vi "Set Steer Motors.vi"(5 "Disable":bool, 6 "PPR":dbl=1024.0, 7 "Offset Encoder Positions":dbl[](array[numeric]), 8 "Steer Control Mode":T2, 9 "Motor List":T1[](array[typedef])=[enum."Right-Front", enum."Left-Front", enum."Left-Back", enum."Right-Back"], 10 "Swerve Data":T8 {"Back Right"."Angle" scale format="%.3f"; "Back Right"."Velocity" scale=-1.0..1.0 scale format="%.1f"; "Back Left"."Angle" scale format="%.3f"; "Back Left"."Velocity" scale=-1.0..1.0 scale format="%.1f"; "Front Left"."Angle" scale format="%.3f"; "Front Left"."Velocity" scale=-1.0..1.0 scale format="%.1f"; "Front Right"."Angle" scale format="%.3f"; "Front Right"."Velocity" scale=-1.0..1.0 scale format="%.1f"}, 11 "Steer Refs":T3[](array[typedef])) -> (1 "Encoder Counts Out":dbl[](array[numeric]), 3 "Array Out":T3[](array[typedef]))   [LabVIEW 2023, in "SwerveDrive_ACT_ts.lvlib"]
uses:
  SwerveDrive_ACT_ts.lvlib
  Shared Code/TypeDefs/Cluster_Swerve 4 Steer and Velocity.ctl
  Shared Code/TypeDefs/Cluster_Module Velocity-Direction-Rotations.ctl
  Shared Code/TypeDefs/Level_Velocity plus-minus 1.ctl
  Shared Code/TypeDefs/Dial_Compase heading unit circle CCW positive.ctl
  <vilib>/Rock Robotics/WPI/MotorControl/WPI_MotorControlDeviceRef.ctl
  <vilib>/Rock Robotics/WPI/MotorControl/WPI_MotorControlType.ctl
  <vilib>/Rock Robotics/SystemInterfaces/DIO/FPGA_DIOPWMChannel.ctl
  <vilib>/Rock Robotics/WPI/PWM/WPI_PWMDeadband.ctl
  <vilib>/Rock Robotics/SystemInterfaces/DIO/FPGA_DIOChannel.ctl
  Type Defs/ENUM_Steer Mode Select.ctl
  Shared Code/TypeDefs/ENUM_Module Position.ctl
  <vilib>/Rock Robotics/WPI/ThirdParty/REV Robotics/REVLib/Typedef/Spark MAX Control Type.ctl
panel:
  # "\"Front\" of Robot"
  # "Index 1"
  # "Index 0"
  # "Index 3"
  # "Index 2"
  # "Right Hand Rule"
  # "X"
  # "+CCW"
  # "Y"
  # "(0,0)"
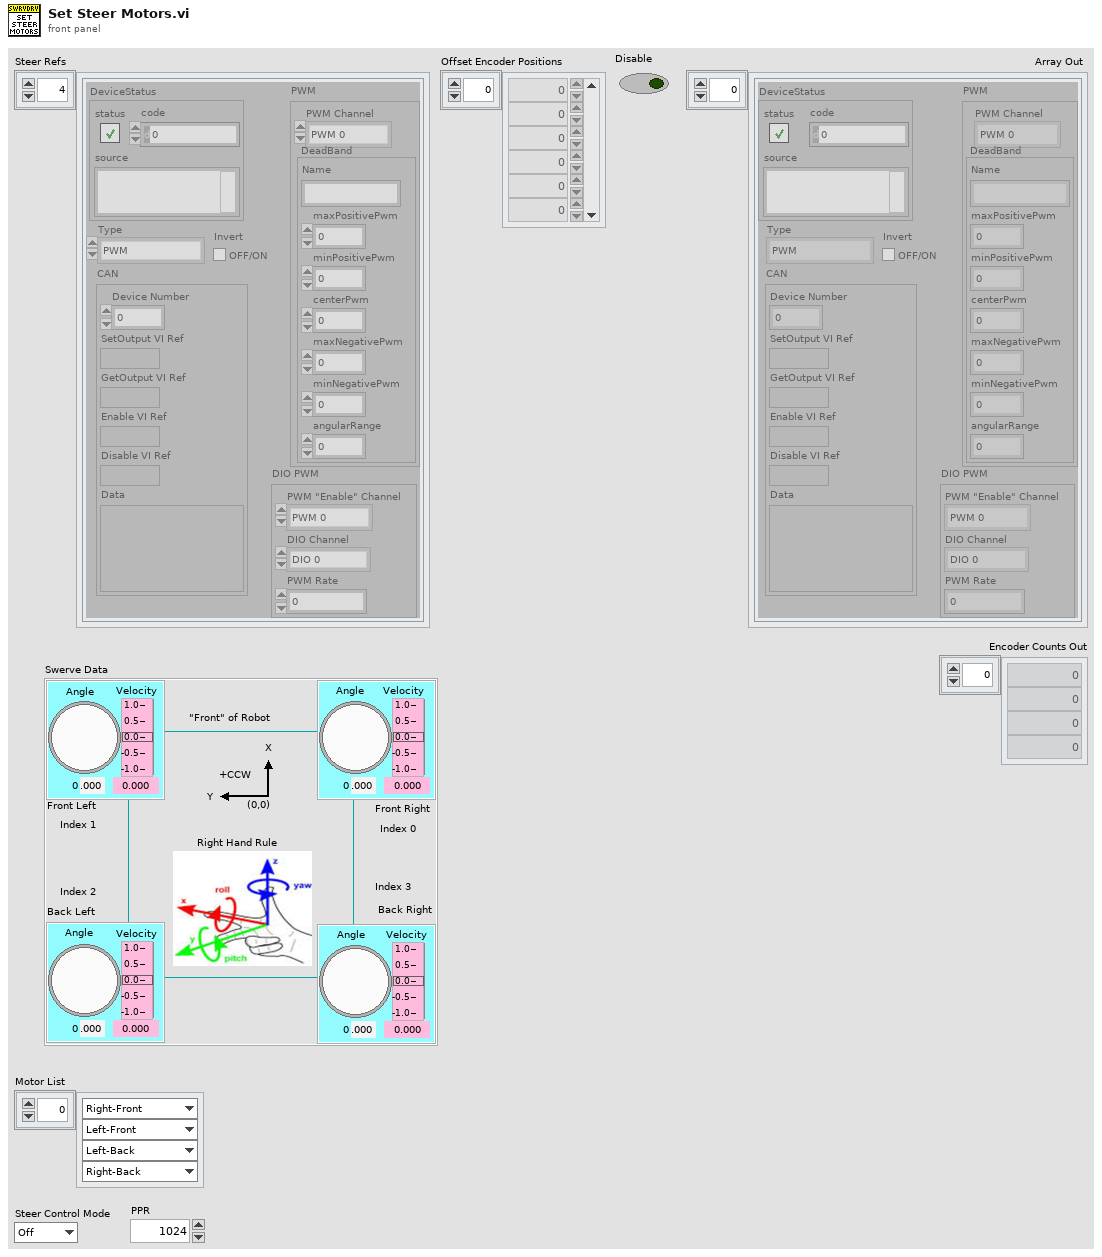
[diagram p1: front panel]
types:
  T1 = typedef "ENUM_Module Position.ctl" = enum16{"Left-Front", "Right-Front", "Left-Back", "Right-Back"}
  T2 = typedef "ENUM_Steer Mode Select.ctl" = enum16{"Off", "Hold", "Steer"}
  T3 = typedef "WPI_MotorControlDeviceRef.ctl" = cluster{"DeviceStatus":errorcluster, "Type":T4, "PWM":cluster{"PWM Channel":T5, "DeadBand":T6}, "CAN":cluster{"Device Number":u8, "SetOutput VI Ref":variant, "GetOutput VI Ref":variant, "Enable VI Ref":variant, "Disable VI Ref":variant, "Data":variant}, "Invert":bool, "DIO PWM":cluster{"PWM \"Enable\" Channel":T5, "DIOChannel":T7, "PWM Rate":dbl}}
  T4 = typedef "WPI_MotorControlType.ctl" = enum16{"PWM", "CAN", "DIO PWM"}
  T5 = typedef "FPGA_DIOPWMChannel.ctl" = enum8{"PWM 0", "PWM 1", "PWM 2", "PWM 3", "PWM 4", "PWM 5", "PWM 6", "PWM 7", "PWM 8", "PWM 9", "PWM MXP 0", "PWM MXP 1", "PWM MXP 2", "PWM MXP 3", "PWM MXP 4", "PWM MXP 5", "PWM MXP 6", "PWM MXP 7", "PWM MXP 8", "PWM MXP 9", "Invalid"}
  T6 = typedef "WPI_PWMDeadband.ctl" = cluster{"Name":string, "maxPositivePwm":i32, "minPositivePwm":i32, "centerPwm":i32, "maxNegativePwm":i32, "minNegativePwm":i32, "angularRange":u16}
  T7 = typedef "FPGA_DIOChannel.ctl" = enum8{"DIO 0", "DIO 1", "DIO 2", "DIO 3", "DIO 4", "DIO 5", "DIO 6", "DIO 7", "DIO 8", "DIO 9", "DIO MXP 0", "DIO MXP 1", "DIO MXP 2", "DIO MXP 3", "DIO MXP 4", "DIO MXP 5", "DIO MXP 6", "DIO MXP 7", "DIO MXP 8", "DIO MXP 9", "DIO MXP 10", "DIO MXP 11", "DIO MXP 12", "DIO MXP 13", "DIO MXP 14", "DIO MXP 15", "SPI Port CS1", "SPI Port CS2", "SPI Port CS3", "SPI Port MISO", "SPI Port MOSI", "Invalid"}
  T8 = typedef "Cluster_Swerve 4 Steer and Velocity.ctl" = cluster{"Front Right":T9, "Front Left":T9, "Back Left":T9, "Back Right":T9}
  T9 = typedef "Cluster_Module Velocity-Direction-Rotations.ctl" = cluster{"Velocity":T10, "Angle":T11, "Rotations Count":dbl}
  T10 = typedef "Level_Velocity plus-minus 1.ctl" = dbl
  T11 = typedef "Dial_Compase heading unit circle CCW positive.ctl" = dbl
  T12 = typedef "Spark MAX Control Type.ctl" = enum16{"Percent VBus", "Voltage", "Velocity", "Position", "Smart Motion", "Current", "Smart Velocity"}
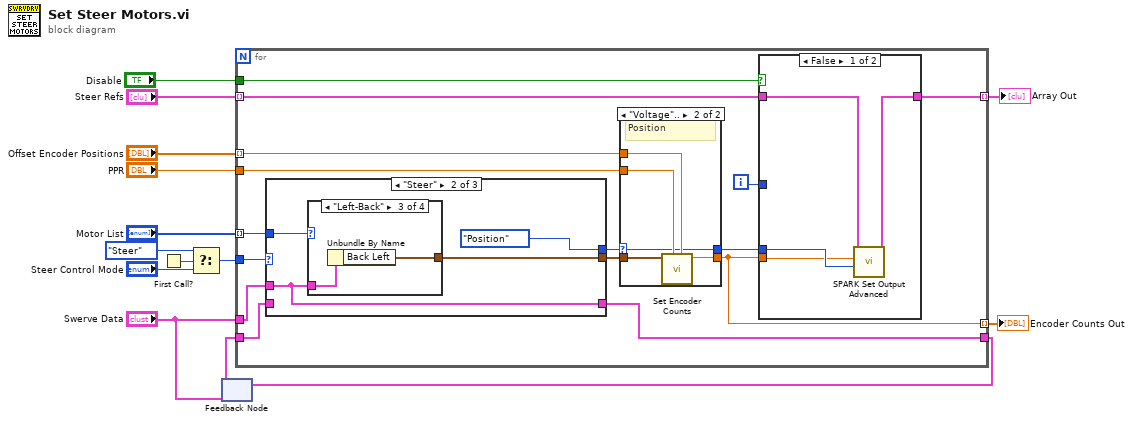
[diagram p0: block diagram]
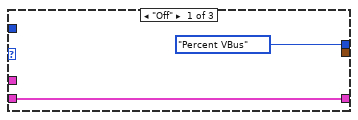
[diagram p3: hidden frame]
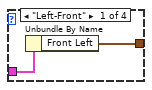
[diagram p4: hidden frame]
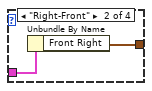
[diagram p5: hidden frame]
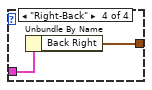
[diagram p6: hidden frame]
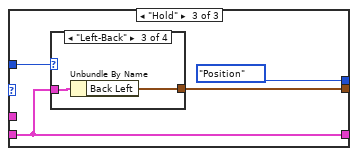
[diagram p7: hidden frame]
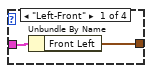
[diagram p8: hidden frame]
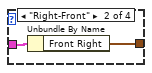
[diagram p9: hidden frame]
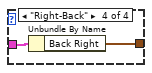
[diagram p10: hidden frame]
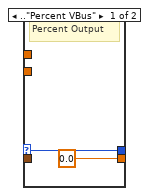
[diagram p11: hidden frame]
diagram:
  n1 = First Call?() -> (First Call?: T/F=w8:bool)
  n2 = Select(t=ENUM_Steer_Mode_Select."Steer" ("Steer Control Mode"), s=w8, f="Steer Control Mode") -> (s? t:f=w5:T2)
  n3 = feedback #1("Swerve Data") -> (w9:T8)
  n4 = for {
    tunnel: "Steer Refs" -> [w29] mode=indexing
    tunnel: "Swerve Data" -> [w26]
    tunnel: [w28] -> w14 mode=indexing
    tunnel: "Offset Encoder Positions" -> [w23] mode=indexing
    tunnel: w5 -> [w27]
    tunnel: "PPR" -> [w24]
    tunnel: "Motor List" -> [w25] mode=indexing
    tunnel: w9 -> [w21]
    tunnel: [w20] -> w3
    tunnel: [w17] -> w2 mode=indexing
    tunnel: "Disable" -> [w16]
    i -> [w15]
    n5 = case shown="\"Steer\"" w27 {
      tunnel: [Spark_MAX_Control_Type."Percent VBus" ("Control Mode") Spark_MAX_Control_Type."Position" ("Control Mode") Spark_MAX_Control_Type."Position" ("Control Mode")] -> w19
      tunnel: w26 -> [_ w38 _]
      tunnel: w25 -> [_ w40 w52]
      tunnel: [_ w39 w51] -> w22
      tunnel: w21 -> [w36 _ w50]
      tunnel: [w36 w38 w50] -> w20
      frame "Off" {
      }
      frame "Steer" {
        n6 = case shown="\"Left-Back\"" w40 {
          tunnel: w38 -> [w42 w44 w46 w48]
          tunnel: [w41 w43 w45 w47] -> w39
          frame "Left-Front" {
            n7 = Unbundle By Name(w42) -> ("Front Left"=w41:T9)
          }
          frame "Right-Front" {
            n8 = Unbundle By Name(w44) -> ("Front Right"=w43:T9)
          }
          frame "Left-Back" {
            n9 = Unbundle By Name(w46) -> ("Back Left"=w45:T9)
          }
          frame "Right-Back" {
            n10 = Unbundle By Name(w48) -> ("Back Right"=w47:T9)
          }
        }
      }
      frame "Hold" {
        n11 = case shown="\"Left-Back\"" w52 {
          tunnel: w50 -> [w54 w56 w58 w60]
          tunnel: [w53 w55 w57 w59] -> w51
          frame "Left-Front" {
            n12 = Unbundle By Name(w54) -> ("Front Left"=w53:T9)
          }
          frame "Right-Front" {
            n13 = Unbundle By Name(w56) -> ("Front Right"=w55:T9)
          }
          frame "Left-Back" {
            n14 = Unbundle By Name(w58) -> ("Back Left"=w57:T9)
          }
          frame "Right-Back" {
            n15 = Unbundle By Name(w60) -> ("Back Right"=w59:T9)
          }
        }
      }
    }
    n16 = case shown="\"Voltage\".." w19 {
      selector: w19 -> [w61 w63]
      tunnel: w22 -> [_ w66]
      tunnel: w24 -> [_ w65]
      tunnel: w23 -> [_ w64]
      tunnel: [0.0 ("Encder Count Set") w67] -> w17
      tunnel: [w61 w63] -> w18
      frame .."Percent VBus" {
        # "Percent Output"
      }
      frame "Voltage".. {
        # "Position"
        n17 = call "Set Encoder Counts.vi"("Encoder Count at Zero"=w64, "PPR"=w65, "Angle(0-1) in"=w66) -> ("Encder Count Set"=w67:dbl)  [unwired: 8 in]
      }
    }
    n18 = case shown="False" w16 {
      tunnel: w29 -> [w31 w34]
      tunnel: [w30 w34] -> w28
      tunnel: w18 -> [w33 _]
      tunnel: w17 -> [w32 _]
      tunnel: w15 -> [_ _]
      frame False {
        n19 = call <vilib>:"SPARK Set Output Advanced.vi"("Control Mode"=w33, "Setpoint"=w32, "MotorControlDevRef"=w31) -> ("MotorControlDevRef"=w30:T3)  [unwired: 7 in, 1 out]
      }
      frame True {
      }
    }
  }
  "Array Out" <- w14
  "Encoder Counts Out" <- w2
  n20 = feedback-in #1(w3) -> ()
